vi "Read VISA resource name.vi"(8 "error in (no error)":errorcluster, 11 "Strain Digitizer in":refnum<class "Strain Digitizer.lvclass">) -> (0 "error out":errorcluster, 2 "VISA resource name":refnum<visa-resource-name>="TCPIP0::192.168.1.69::1852::SOCKET", 3 "Strain Digitizer out":refnum<class "Strain Digitizer.lvclass">)   [LabVIEW 2015, in "Strain Digitizer.lvclass"]
uses:
  Strain Digitizer.lvclass
  Strain Digitizer.lvclass/Strain Digitizer.ctl
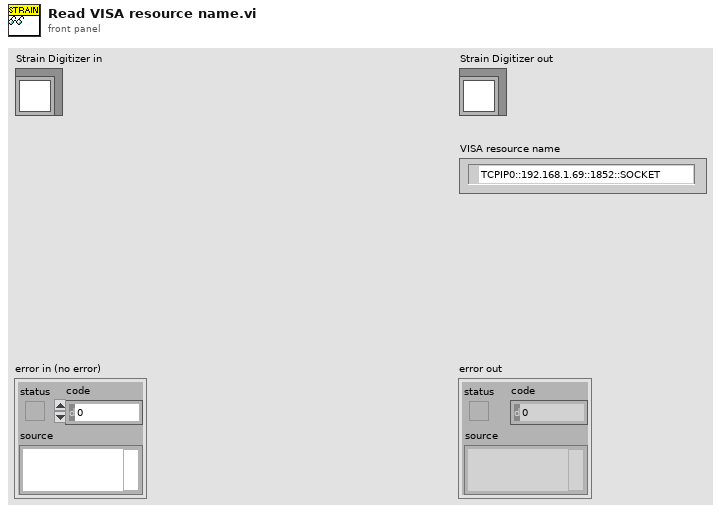
[diagram p1: front panel]
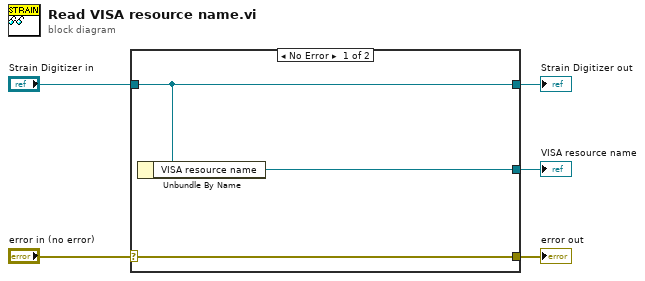
[diagram p0: block diagram]
diagram:
  n1 = case shown="No Error" "error in (no error)" {
    selector: "error in (no error)" -> [w8 w9]
    tunnel: [w8 w9] -> w4
    tunnel: [w7 w10] -> w2
    tunnel: "Strain Digitizer in" -> [w7 w10]
    tunnel: [w6 _] -> w1
    frame No Error {
      n2 = Unbundle By Name(w7) -> ("VISA resource name"=w6:refnum<visa-resource-name>)
    }
    frame Error {
    }
  }
  "error out" <- w4
  "Strain Digitizer out" <- w2
  "VISA resource name" <- w1
